vi "Gradient Update.vi"(8 "Learning Rate":dbl=0.007 format="%#_13g", 10 "Error":dbl, 11 "Phi":dbl[](array[numeric])) -> (3 "Gradient Update":dbl[](array[numeric]))   [LabVIEW 2021]
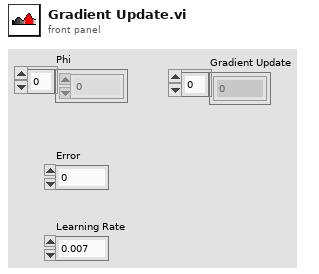
[diagram p1: front panel]
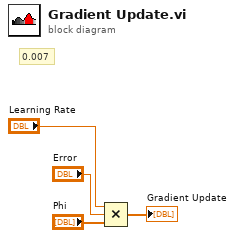
[diagram p0: block diagram]
diagram:
  # "0.007"
  n1 = Compound Arithmetic op=MULTIPLY("Learning Rate", "Error", "Phi") -> (→"Gradient Update":dbl[])
